vi "VerifySignature.vi"(5 "RSASignPadding":T2, 7 "HashingAlgorithm":T1=enum."SHA512", 8 "error in (no error)":errorcluster, 9 "Signature in":u8[](array[numeric]), 10 "Data in":u8[](array[numeric]), 11 "CngKey in":refnum<k24>) -> (0 "error out":errorcluster, 2 "Verified?":bool, 3 "CngKey out":refnum<k24>)   [LabVIEW 2021, in "dotNET Crypto Asymmetric Encryption.lvlib"]
doc: "Verify the signature of the data using the public key."
uses:
  RSASignaturePadding.ctl
  HashingAlgorithm.ctl
  System.Core
  dotNET Crypto Asymmetric Encryption.lvlib
  Utility/dotNET Crypto Utility.lvlib
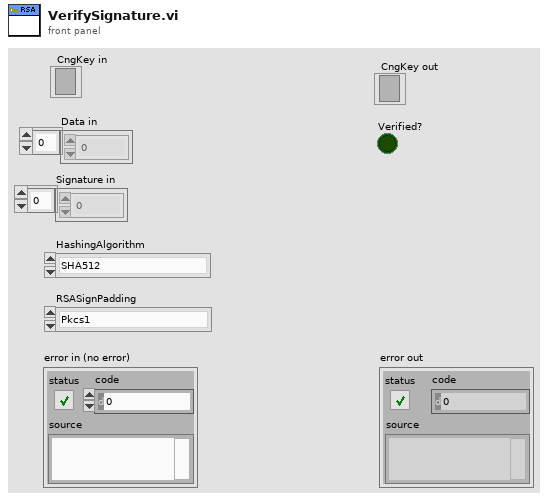
[diagram p1: front panel]
types:
  T1 = typedef "dotNET Crypto Utility.lvlib/HashingAlgorithm.ctl" = enum16{"MD5", "SHA1", "SHA256", "SHA384", "SHA512"}
  T2 = typedef "dotNET Crypto Asymmetric Encryption.lvlib/RSASignaturePadding.ctl" = enum16{"Pkcs1", "Pss"}
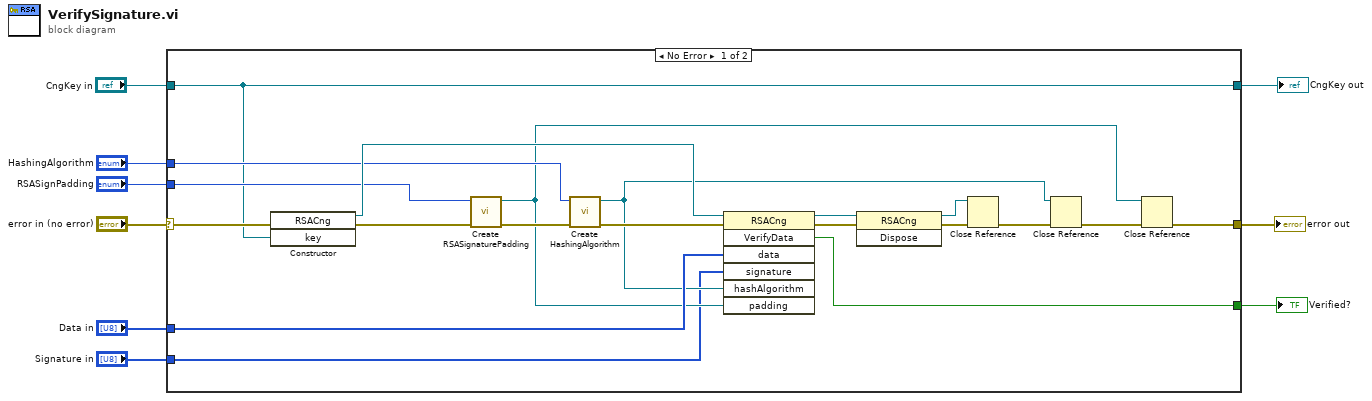
[diagram p0: block diagram]
diagram:
  n1 = case shown="No Error" "error in (no error)" {
    selector: "error in (no error)" -> [w11 w31]
    tunnel: "Data in" -> [w29 _]
    tunnel: "RSASignPadding" -> [w22 _]
    tunnel: "HashingAlgorithm" -> [w17 _]
    tunnel: [w14 _] -> w6
    tunnel: "Signature in" -> [w13 _]
    tunnel: [w12 w31] -> w4
    tunnel: "CngKey in" -> [w10 w30]
    tunnel: [w10 w30] -> w1
    frame No Error {
      n2 = constructor class="RSACng"(error in=w11, "key"=w10) -> (reference out=w23:refnum<k24>, error out=w24:errorcluster)  [unwired: 2 in, 2 out]
      n3 = call "Create RSASignaturePadding.vi"("error in (no error)"=w24, "RSASignaturePadding"=w22) -> ("error out"=w21:errorcluster, "RSASignaturePadding out"=w16:refnum<k24>)  [unwired: 8 in]
      n4 = call "Create HashingAlgorithm.vi"("error in (no error)"=w21, "HashingAlgorithm"=w17) -> ("error out"=w20:errorcluster, "Hashing Algorithm"=w15:refnum<k24>)  [unwired: 8 in]
      n5 = invoke class="RSACng" method="VerifyData"(reference=w23, error in=w20, "data"=w29, "signature"=w13, "hashAlgorithm"=w15, "padding"=w16) -> (reference out=w27:refnum<k24>, error out=w28:errorcluster, "VerifyData"=w14:bool)  [unwired: 1 in, 4 out]
      n6 = invoke class="RSACng" method="Dispose"(reference=w27, error in=w28) -> (reference out=w26:refnum<k24>, error out=w25:errorcluster)  [unwired: 1 in, 1 out]
      n7 = Close Reference(reference=w26, error in (no error)=w25) -> (error out=w19:errorcluster)
      n8 = Close Reference(reference=w15, error in (no error)=w19) -> (error out=w18:errorcluster)
      n9 = Close Reference(reference=w16, error in (no error)=w18) -> (error out=w12:errorcluster)
    }
    frame Error {
    }
  }
  "error out" <- w4
  "Verified?" <- w6
  "CngKey out" <- w1
